vi "Count Command Errors.vi"(8 "Error In":errorcluster) -> (0 "Error Out":errorcluster, 3 "Command Errors":i32)   [LabVIEW 2019]
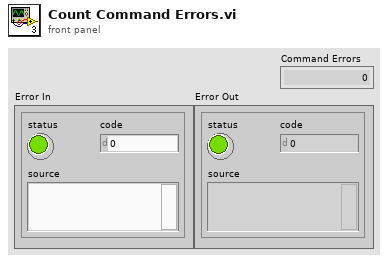
[diagram p1: front panel]
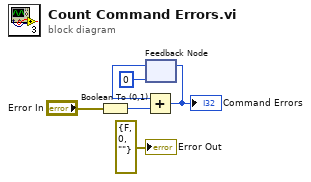
[diagram p0: block diagram]
diagram:
  n1 = Boolean To (0,1)(Boolean="Error In") -> (0, 1=w6:i16)
  n2 = feedback #1(0) -> (w4:i32)
  n3 = Add(x=w4, y=w6) -> (x+y=w5:i32)
  "Command Errors" <- w5
  n4 = feedback-in #1(w5) -> ()
  "Error Out" <- errorcluster {"status"=FALSE, "code"=0, "source"=""} ("Error Out")
